vi "Write Encoder Position.vi"(10 "Encoder Position":dbl[unit], 11 "StiffnessMonitor in":refnum<class "StiffnessMonitor.lvclass">) -> (3 "StiffnessMonitor out":refnum<class "StiffnessMonitor.lvclass">)   [LabVIEW 2013, in "StiffnessMonitor.lvclass"]
uses:
  StiffnessMonitor.lvclass
  StiffnessMonitor.lvclass/StiffnessMonitor.ctl
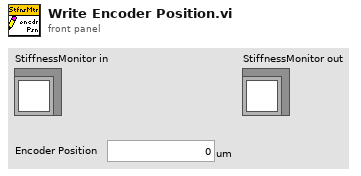
[diagram p1: front panel]
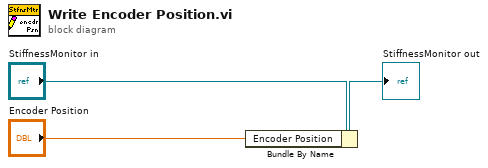
[diagram p0: block diagram]
diagram:
  n1 = Bundle By Name(cluster="StiffnessMonitor in", "Encoder Position"="Encoder Position") -> (→"StiffnessMonitor out":refnum<class "StiffnessMonitor.lvclass">)
